vi "AutomatedStart_Flo.vi"() -> ()   [LabVIEW 2014]
uses:
  <vilib>/userdefined/High Color/nirio_resource_hc.ctl
  TriggerChannel.ctl
  <vilib>/FPGAPlugInAG/PCI-7813R/niLvFpga_Open_PCI-7813R.vi
  <vilib>/rvi/interface/nirviOpenFPGA/nirviOpenFPGA.xnode
  FPGA Bitfiles/W7XBolo2017_FPGATarget_fmain2014_DACRangeVoltage.lvbitx
  f_main_2014.vi
  <vilib>/rvi/interface/nirviMethod/nirviMethod.xnode
  <vilib>/FPGAPlugInAG/PCI-7813R/niLvFpga_Reset_PCI-7813R.vi
panel:
  in  "Reset FPGA after?":bool
  out "Operation Watchdog":bool
  out "No. of Software Triggers \ndetected":dbl
  out "No. of Hardware Triggers \ndetected":dbl
  out "Autmated Start Loop Counter \n(Increasing every 1s)":i32
  out "Timeout ? \n(1s-10s?)":bool
  out "Hardware Trigger \ndetected":bool
  in  "Software Trigger\n(Switch until released)":bool
  in  "Stopp Button":bool
  # "Automated Start W7-X Bolometer DAQ"
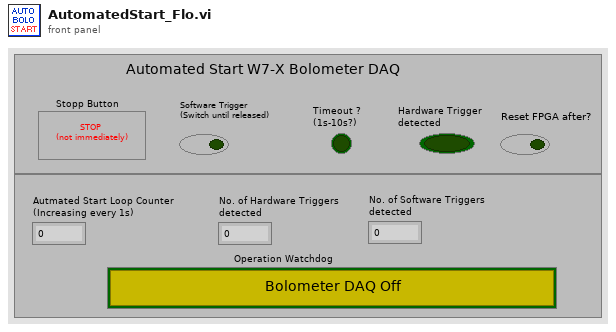
[diagram p1: front panel]
types:
  T1 = typedef "TriggerChannel.ctl" = enum16{"board0 (broken)", "board1 (t = -60sec)", "board2 (t = 0sec)"}
  T2 = enum32{"Invalid", "Standard", "Closed", "Hidden", "Minimized", "Maximized"}
  T3 = typedef "nirio_resource_hc.ctl" = tag
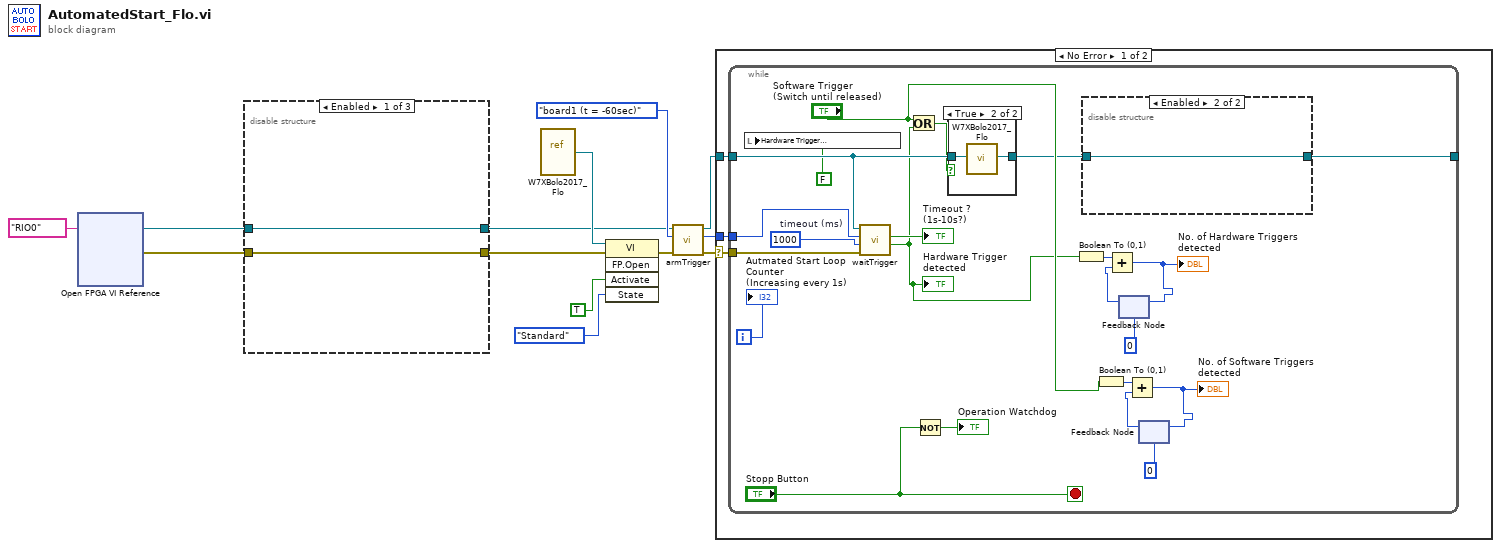
[diagram p0: block diagram]
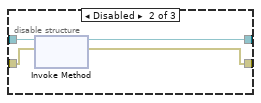
[diagram p2: hidden frame]
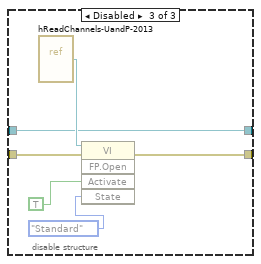
[diagram p3: hidden frame]
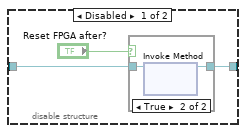
[diagram p4: hidden frame]
diagram:
  n1 = xnode "Open FPGA VI Reference"("resource name"=T3 "RIO0") -> ("FPGA VI Reference Out"=w3:refnum<k20>, "error out"=w1:errorcluster)  [unwired: 1 in]
  n2 = disable-structure shown="Enabled" {
    disable-tunnel: [w15 w17 w21] -> w4
    disable-tunnel: w3 -> [w15 w19 w21]
    disable-tunnel: w1 -> [w14 w18 w22]
    disable-tunnel: [w14 w16 w20] -> w2
    frame Enabled {
    }
    frame Disabled {
      n3 = xnode "Invoke Method"("FPGA VI Reference In"=w19, "error in"=w18) -> ("FPGA VI Reference Out"=w17:refnum<k20>, "error out"=w16:errorcluster)
    }
    frame Disabled {
      n4 = vi-ref "hReadChannels-UandP-2013.vi"() -> (w23:refnum<vi>)
      n5 = invoke class="VI" method="FP.Open"(reference=w23, error in=w22, "Activate"=TRUE ("Activate?"), "State"=T2."Standard") -> (error out=w20:errorcluster)  [unwired: 1 in, 4 out]
    }
  }
  n6 = vi-ref "W7XBolo2017_Flo.vi"() -> (w5:refnum<vi>)
  n7 = invoke class="VI" method="FP.Open"(reference=w5, error in=w2, "Activate"=TRUE ("Activate?"), "State"=T2."Standard") -> (error out=w10:errorcluster)  [unwired: 1 in, 4 out]
  n8 = call "armTrigger.vi"("error in (no error)"=w10, "Trigger default: board0 (t = 0)"=TriggerChannel."board1 (t = -60sec)", "Refnum in"=w4) -> ("error out"=w9:errorcluster, "IRQ"=w6:i32, "Refnum out"=w7:refnum<k20>)  [unwired: 6 in]
  n9 = case shown="No Error" w9 {
    selector: w9 -> [w26 _]
    tunnel: w7 -> [w28 _]
    tunnel: w6 -> [w27 _]
    frame No Error {
      n10 = while {
        tunnel: w27 -> [w48]
        tunnel: w26 -> [w47]
        tunnel: w28 -> [w50]
        tunnel: [w29] -> _
        i -> [w44]
        stop <- "Stopp Button" stop-if-true
        w49 = 1000  # timeout (ms)
        n11 = local write "Hardware Trigger \ndetected"(FALSE) -> ()
        n12 = call "waitTrigger.vi"("error in (no error)"=w47, "timeout (ms) default: 10s"=w49, "IRQ"=w48, "Refnum in"=w50) -> ("Boolean"=w33:bool, "Timed Out"=→"Timeout ? \n(1s-10s?)":bool)  [unwired: 4 in, 2 out]
        "Hardware Trigger \ndetected" <- w33
        n13 = Or(x="Software Trigger\n(Switch until released)", y=w33) -> (x .or. y?=w39:bool)
        n14 = Not(x="Stopp Button") -> (.not. x?=→"Operation Watchdog":bool)
        n15 = case shown="True" w39 {
          tunnel: w50 -> [w58 w60]
          tunnel: [w58 w59] -> w30
          frame False {
          }
          frame True {
            n16 = call "W7XBolo2017_Flo.vi"("FPGA VI\nReference In"=w60) -> ("FPGA VI Reference Out"=w59:refnum<k20>)
          }
        }
        n17 = Boolean To (0,1)(Boolean=w33) -> (0, 1=w42:i16)
        n18 = disable-structure shown="Enabled" {
          disable-tunnel: w30 -> [w53 w57]
          disable-tunnel: [w52 w57] -> w29
          frame Disabled {
            n19 = case shown="True" "Reset FPGA after?" {
              tunnel: w53 -> [w54 w56]
              tunnel: [w54 w55] -> w52
              frame False {
              }
              frame True {
                n20 = xnode "Invoke Method"("FPGA VI Reference In"=w56) -> ("FPGA VI Reference Out"=w55:refnum<k20>)  [unwired: 1 in, 1 out]
              }
            }
          }
          frame Enabled {
          }
        }
        n21 = Boolean To (0,1)(Boolean="Software Trigger\n(Switch until released)") -> (0, 1=w37:i16)
        n22 = feedback #1(i16 0) -> (w43:i16)
        n23 = Add(x=w42, y=w43) -> (x+y=w40:i16)
        "No. of Hardware Triggers \ndetected" <- w40
        n24 = feedback-in #1(w40) -> ()
        n25 = feedback #2(i16 0) -> (w38:i16)
        n26 = Add(x=w37, y=w38) -> (x+y=w35:i16)
        "No. of Software Triggers \ndetected" <- w35
        n27 = feedback-in #2(w35) -> ()
        "Autmated Start Loop Counter \n(Increasing every 1s)" <- w44
      }
    }
    frame Error {
    }
  }
